vi "BRig_dataBlock_c_nTrial.vi"() -> (2 "output_c_nTrial":i32)   [LabVIEW 2014]
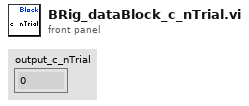
[diagram p1: front panel]
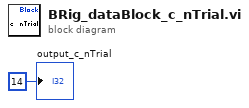
[diagram p0: block diagram]
diagram:
  "output_c_nTrial" <- 14 ("output_iBlock")
